vi "09 main.vi"() -> ()   [LabVIEW 2020]
panel:
  in  "Animate?":bool
  out "Unique visits":i32
  out "2D Picture":picture
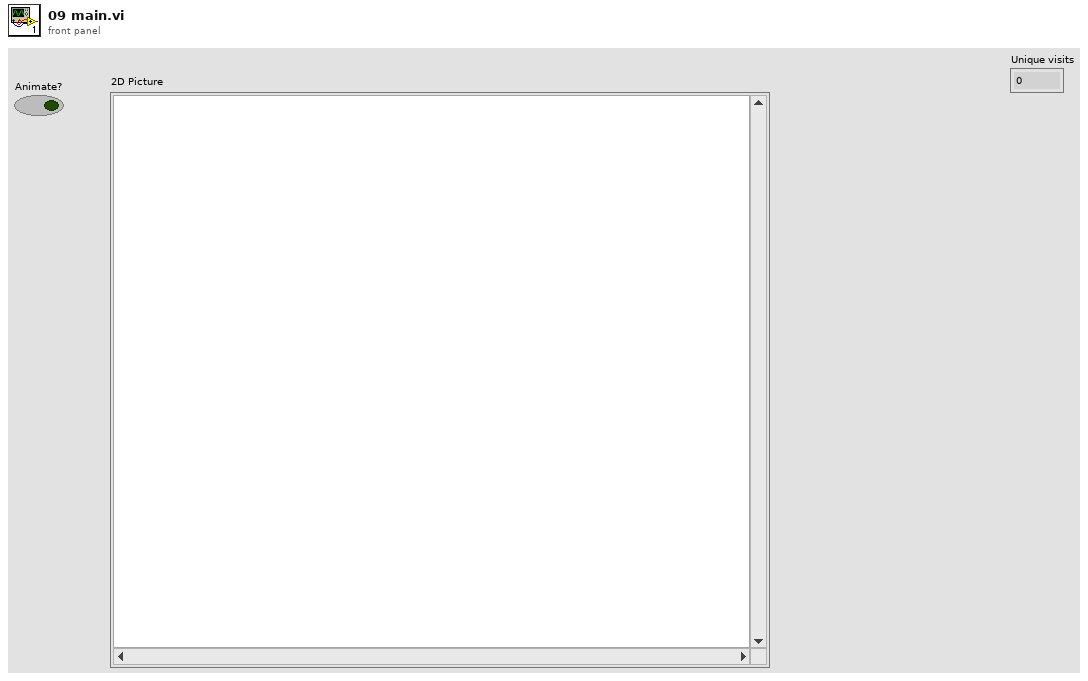
[diagram p1: front panel]
types:
  T1 = cluster{"left":i16, "top":i16, "right":i16, "bottom":i16}
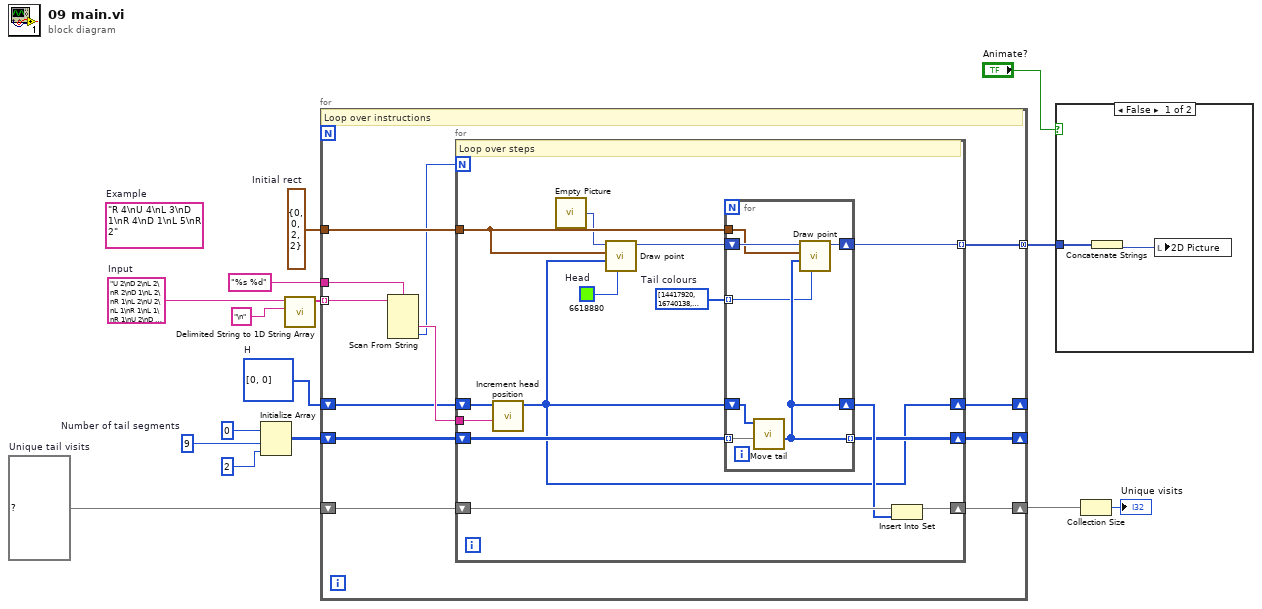
[diagram p0: block diagram]
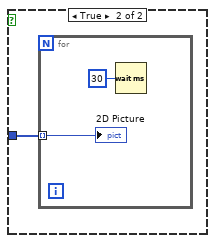
[diagram p2: hidden frame]
diagram:
  w12 = T1 {"left"=0, "top"=0, "right"=2, "bottom"=2}  # Initial rect
  w6 = 9  # Number of tail segments
  w11 = set{i32[]} {}  # Unique tail visits
  w8 = i32[] [0, 0]  # H
  w3 = "U 2\nD 2\nL 2\nR 2\nD 1\nL 2\nR 1\nL 2\nU 2\nL 1\nR 1\nL 1\nR 1\nU 2\nD 2\nL 1\nU 1\nL 2\nD 1\nU 2\nD 1\nR 1\nD 1\nU 2\nD 2\nU 1\nR 2\nD 2\nR 1\nU 1\nD 1\nR 1\nL 2\nU 2\nD 2\nL 1\nR 2\nL 2\nR 1\nD 1\nR 1\nD 2\nU 2\nR 2\nD 2\nU 2\nD 1\nU 1\nR 2\nU 2\nR 2\nU 2\nD 1\nU 1\nR 2\nD 1\nU 2\nL 1\nU 2\nD 1\nR 2\nU 1\nR 2\nD 1\nL 2\nR 1\nL 1\nR 2\nU 1\nL 1\nD 2\nL 2\nD 1\nR 2\nD 1\nR 2\nU 1\nD 1\nL 1\nR 1\nL 2\nR 1\nU 1\nD 2\nL 1\nD 2\nR 1\nL 1\nR 1\nU 2\nL 2\nD 1\nU 1\nD 2\nU 2\nR 2\nU 2\nR 1\nU 2\nD 1\nR 2\nD 2\nU 1\nD 1\nR 2\nU 1\nR 2\nL 1\nR 1\nD 2\nU 1\nR 3\nD 1\nR 1\nL 3\nD 2\nR 1\nD 1\nR 3\nL 2\nD 2\nL 1\nU 3\nD 3\nL 1\nD 1\nL 3\nD 1\nU 3\nL 1\nR 2\nU 2\nD 1\nL 2\nD 3\nR 1\nU 2\nL 2\nU 1\nL 1\nU 2\nD 2\nU 1\nL 1\nD 3\nR 1\nD 3\nR 1\nD 1\nU 1\nL 2\nU 3\nD 2\nU 1\nR 3\nD 1\nU 3\nL 3\nU 1\nR 2\nL 2\nR 1\nL 1\nU 1\nL 1\nD 2\nL 2\nU 2\nL 1\nD 2\nR 1\nU 2\nL 2\nR 2\nL 1\nU 2\nL 2\nR 3\nL 3\nD 1\nR 3\nL 3\nD 2\nU 3\nL 3\nD 2\nR 2\nL 2\nD 2\nU 2\nL 3\nR 1\nU 2\nL 1\nD 3\nU 2\nD 3\nL 2\nD 3\nU 1\nD 3\nU 3\nL 3\nD 2\nL 3\nR 2\nD 3\nR 1\nD 2\nU 2\nD 1\nU 3\nD 2\nL 2\nD 1\nR 1\nL 2\nR 2\nL 3\nU 3\nL 1\nD 2\nR 1\nL 2\nD 2\nR 1\nD 1\nL 4\nD 2\nR 3\nU 4\nR 4\nU 1\nD 4\nU 4\nD 4\nU 2\nR 3\nU 3\nR 4\nU 3\nL 2\nR 1\nU 4\nD 4\nR 2\nD 4\nR 2\nU 2\nD 1\nR 1\nL 3\nR 2\nD 3\nR 3\nU 1\nD 2\nR 4\nU 1\nD 4\nR 1\nU 1\nD 2\nU 4\nD 3\nL 1\nD 4\nL 2\nD 2\nR 3\nL 1\nU 4\nL 4\nU 3\nD 3\nL 2\nD 3\nU 1\nR 4\nD 3\nL 3\nD 4\nL 1\nD 2\nU 4\nL 2\nD 1\nR 3\nD 4\nU 3\nD 4\nU 2\nL 2\nR 3\nL 4\nR 2\nL 4\nU 3\nL 4\nD 3\nU 4\nL 2\nU 3\nR 2\nD 2\nU 1\nD 2\nL 1\nR 4\nD 3\nL 1\nD 3\nU 2\nL 4\nD 4\nL 4\nR 3\nL 3\nU 2\nL 1\nR 2\nL 4\nD 2\nL 3\nU 3\nD 1\nL 2\nR 3\nU 4\nR 1\nU 3\nD 4\nL 2\nU 2\nL 2\nR 5\nD 5\nU 3\nR 4\nL 4\nU 5\nD 3\nU 2\nL 5\nU 1\nR 3\nL 3\nU 4\nL 3\nD 5\nU 2\nR 1\nU 4\nR 5\nD 2\nL 1\nU 3\nR 5\nD 2\nU 3\nD 5\nU 2\nD 2\nU 2\nL 4\nU 5\nR 4\nU 4\nL 3\nU 5\nR 4\nL 4\nD 5\nR 4\nD 4\nL 2\nR 3\nL 5\nD 3\nU 2\nD 4\nR 1\nU 5\nR 4\nD 1\nU 1\nL 1\nU 3\nD 2\nU 4\nD 3\nU 5\nR 2\nU 5\nL 1\nR 5\nU 5\nR 4\nD 3\nR 1\nD 3\nU 3\nR 1\nL 1\nD 5\nU 4\nR 3\nD 3\nL 2\nU 1\nL 2\nU 5\nD 5\nU 2\nD 4\nL 2\nD 2\nL 1\nD 4\nU 2\nD 4\nR 1\nU 1\nD 4\nL 3\nD 3\nU 2\nD 2\nL 1\nD 5\nR 1\nL 2\nD 5\nU 5\nL 3\nD 1\nR 2\nL 2\nU 1\nL 2\nD 5\nL 1\nR 2\nD 4\nU 6\nL 4\nR 5\nD 4\nU 2\nR 1\nD 4\nL 2\nR 5\nL 6\nR 2\nU 6\nR 5\nD 1\nU 1\nL 6\nR 2\nL 6\nD 3\nL 2\nR 6\nU 6\nL 1\nD 3\nR 1\nD 2\nR 4\nL 4\nU 6\nL 3\nD 1\nU 1\nL 4\nR 3\nD 3\nR 6\nD 3\nL 4\nR 5\nL 5\nD 3\nU 3\nD 6\nR 4\nD 5\nL 2\nD 1\nR 4\nL 6\nR 5\nU 4\nD 5\nL 3\nD 1\nL 6\nD 5\nL 3\nU 3\nR 4\nL 4\nD 6\nR 3\nL 1\nR 1\nU 4\nD 6\nL 3\nR 2\nD 1\nL 2\nU 3\nD 3\nL 5\nU 6\nL 5\nD 5\nR 5\nU 6\nD 2\nU 2\nR 5\nU 6\nD 2\nR 1\nL 3\nU 1\nL 6\nU 1\nR 3\nL 3\nD 4\nU 2\nR 3\nL 1\nD 3\nR 5\nL 2\nD 3\nL 2\nU 6\nR 5\nU 5\nL 1\nU 5\nL 6\nD 4\nU 2\nL 5\nU 3\nD 2\nU 4\nD 4\nU 2\nR 5\nL 4\nD 3\nR 6\nD 1\nR 4\nU 5\nL 7\nD 2\nR 6\nU 4\nL 5\nD 5\nL 2\nD 1\nR 4\nD 6\nL 5\nD 4\nR 7\nU 4\nD 7\nU 4\nR 3\nL 7\nR 7\nD 3\nR 5\nU 2\nR 3\nD 5\nR 5\nU 4\nD 2\nU 5\nR 1\nU 5\nR 5\nU 7\nR 4\nD 6\nL 1\nU 3\nD 4\nU 3\nD 7\nU 2\nL 4\nD 6\nR 7\nU 1\nL 6\nD 4\nR 6\nD 4\nU 5\nL 4\nD 6\nL 5\nD 1\nL 5\nU 3\nL 3\nU 2\nR 6\nU 3\nD 4\nU 4\nL 1\nD 3\nL 3\nR 6\nU 2\nL 3\nD 7\nL 2\nU 7\nL 4\nU 4\nD 7\nL 4\nD 3\nL 3\nD 3\nU 1\nD 5\nL 1\nR 4\nD 7\nL 7\nD 6\nR 3\nU 1\nR 6\nL 4\nD 6\nR 5\nU 7\nL 6\nR 6\nL 3\nD 4\nU 1\nR 2\nL 1\nR 1\nU 4\nD 1\nL 4\nR 2\nU 4\nR 3\nD 1\nU 3\nR 4\nL 2\nU 4\nL 3\nD 7\nR 6\nU 4\nL 4\nD 7\nR 6\nD 7\nL 5\nR 5\nD 7\nR 4\nD 1\nL 6\nU 8\nL 4\nU 2\nL 6\nR 1\nL 5\nU 5\nD 3\nL 8\nR 3\nL 3\nR 5\nU 4\nR 6\nD 4\nU 1\nL 2\nR 8\nD 7\nU 3\nD 4\nL 8\nU 6\nL 5\nR 1\nU 1\nR 4\nU 5\nD 2\nR 2\nU 2\nL 1\nU 8\nD 4\nR 7\nU 3\nD 6\nR 6\nL 3\nR 8\nD 7\nU 2\nR 5\nL 3\nU 1\nD 6\nR 1\nD 3\nL 2\nU 2\nD 8\nU 8\nL 8\nU 5\nD 6\nU 6\nL 6\nU 6\nD 5\nR 8\nL 7\nD 6\nR 1\nD 4\nL 1\nU 7\nR 3\nL 2\nD 6\nR 6\nD 7\nL 6\nU 5\nR 4\nD 7\nU 7\nD 5\nL 4\nR 6\nD 3\nL 6\nU 2\nD 7\nR 7\nU 5\nD 3\nU 2\nL 1\nD 2\nU 4\nL 1\nR 3\nL 6\nU 9\nD 8\nL 3\nR 3\nD 4\nR 3\nU 6\nL 7\nD 8\nR 9\nD 1\nL 3\nR 6\nD 4\nL 3\nU 6\nL 7\nR 7\nU 9\nL 9\nR 7\nU 8\nR 7\nU 7\nD 1\nL 9\nR 6\nU 4\nD 6\nL 8\nR 7\nD 6\nU 5\nR 6\nD 8\nL 2\nD 5\nR 9\nU 9\nL 7\nU 2\nR 7\nL 6\nU 6\nD 5\nL 8\nD 7\nL 8\nD 9\nR 7\nL 5\nD 9\nL 7\nR 2\nL 6\nR 9\nD 8\nR 8\nU 7\nR 4\nL 6\nR 1\nU 9\nD 2\nR 7\nD 5\nR 4\nD 1\nU 7\nD 5\nR 4\nU 2\nD 5\nL 9\nR 6\nU 7\nD 5\nU 4\nD 6\nL 3\nR 6\nU 3\nR 9\nL 9\nU 4\nD 1\nU 3\nR 7\nD 8\nR 9\nU 1\nR 1\nU 4\nD 7\nR 1\nL 1\nR 8\nD 1\nU 1\nL 3\nU 2\nD 6\nR 6\nL 1\nR 9\nL 2\nD 3\nU 8\nD 9\nU 1\nL 10\nU 10\nD 8\nU 9\nL 3\nR 2\nD 3\nU 4\nL 2\nR 10\nL 9\nU 5\nL 5\nD 4\nL 7\nU 1\nL 1\nR 1\nL 7\nD 7\nU 7\nL 3\nU 10\nR 7\nU 9\nL 6\nR 2\nD 9\nL 10\nD 9\nL 9\nR 5\nL 5\nR 8\nD 9\nR 1\nD 6\nL 1\nU 9\nR 3\nL 10\nD 10\nL 5\nD 10\nR 3\nU 7\nD 6\nU 7\nD 3\nR 5\nD 5\nL 6\nD 4\nU 7\nD 7\nR 9\nU 10\nR 4\nU 1\nR 1\nU 8\nR 3\nU 10\nR 6\nL 1\nU 3\nR 9\nU 2\nD 8\nR 5\nD 3\nR 3\nU 9\nR 6\nL 8\nR 2\nL 5\nR 2\nL 10\nD 2\nL 3\nU 1\nD 10\nL 5\nR 10\nD 7\nL 2\nR 7\nU 6\nD 4\nL 8\nD 8\nU 3\nR 2\nU 10\nD 8\nU 7\nD 9\nU 4\nR 9\nL 2\nR 8\nU 9\nR 10\nU 10\nD 8\nR 8\nU 2\nL 7\nU 3\nL 1\nD 7\nR 1\nU 2\nR 8\nU 4\nD 4\nL 2\nU 9\nL 7\nD 7\nL 2\nR 2\nD 9\nL 11\nU 4\nL 3\nD 7\nU 7\nR 6\nD 7\nU 11\nR 4\nL 3\nR 2\nU 9\nL 1\nU 11\nD 7\nR 10\nD 10\nU 7\nL 1\nU 8\nL 2\nD 11\nL 6\nD 1\nL 8\nD 9\nU 9\nR 5\nL 4\nD 7\nU 8\nL 5\nD 3\nR 6\nL 5\nR 7\nL 7\nD 7\nL 10\nU 4\nL 1\nU 9\nD 2\nR 2\nU 4\nD 3\nR 9\nD 11\nU 10\nL 3\nR 9\nU 6\nL 1\nR 9\nL 8\nU 2\nL 3\nU 9\nD 2\nL 4\nD 5\nU 4\nL 5\nD 11\nL 6\nU 10\nD 9\nU 3\nL 9\nU 11\nD 3\nL 7\nD 4\nL 8\nU 5\nD 10\nL 7\nU 10\nL 10\nU 4\nD 10\nL 7\nR 2\nD 3\nL 6\nR 5\nU 11\nD 4\nU 6\nD 9\nR 2\nL 9\nU 9\nR 11\nU 9\nL 10\nR 8\nL 5\nR 2\nL 12\nR 8\nU 10\nR 7\nD 7\nU 3\nL 10\nU 10\nL 11\nU 1\nR 8\nD 4\nR 3\nD 7\nU 9\nL 2\nR 9\nL 8\nR 6\nL 7\nD 11\nU 12\nD 6\nU 7\nL 11\nD 1\nU 9\nR 7\nL 3\nD 3\nU 5\nR 5\nL 3\nR 11\nL 2\nU 9\nD 9\nR 8\nU 7\nD 5\nL 9\nD 2\nL 1\nR 5\nU 9\nR 10\nU 12\nL 9\nD 12\nR 5\nU 2\nL 7\nR 6\nL 1\nU 12\nL 10\nR 11\nD 1\nL 8\nU 6\nD 10\nR 10\nL 1\nU 11\nD 2\nR 6\nU 1\nR 4\nD 1\nR 6\nU 12\nD 1\nL 1\nU 4\nD 4\nU 12\nD 12\nL 5\nR 10\nD 4\nR 1\nD 8\nU 6\nR 7\nD 12\nU 9\nD 6\nU 6\nD 1\nR 2\nL 7\nR 5\nL 4\nU 1\nL 10\nR 8\nL 12\nD 11\nU 2\nL 10\nD 12\nR 9\nD 1\nU 7\nL 5\nD 4\nU 12\nL 12\nD 11\nU 11\nL 6\nD 2\nR 11\nL 1\nU 10\nL 12\nD 11\nR 8\nD 2\nL 10\nR 4\nL 10\nD 13\nL 10\nD 5\nU 9\nL 3\nD 2\nU 3\nD 11\nL 7\nD 11\nU 4\nD 11\nU 8\nL 5\nU 6\nL 3\nU 3\nR 8\nD 10\nR 1\nD 13\nL 7\nD 7\nR 1\nD 2\nL 3\nD 5\nR 5\nL 5\nU 7\nL 4\nD 1\nL 11\nR 10\nU 8\nD 9\nU 8\nR 11\nL 1\nR 6\nD 6\nU 4\nL 2\nD 11\nU 10\nD 4\nL 11\nR 5\nU 2\nD 10\nU 12\nL 12\nD 11\nL 12\nD 10\nL 4\nU 7\nD 1\nR 4\nL 10\nD 9\nR 5\nD 3\nL 3\nD 5\nR 9\nD 10\nL 8\nR 6\nD 4\nU 5\nR 11\nU 13\nR 10\nU 11\nR 9\nU 4\nD 8\nU 4\nD 6\nR 12\nU 12\nR 9\nU 12\nL 13\nU 6\nD 10\nR 2\nL 5\nU 3\nL 8\nR 11\nD 13\nR 6\nU 13\nL 3\nU 3\nD 4\nL 11\nU 14\nD 13\nU 1\nL 8\nU 13\nR 14\nU 2\nL 13\nR 1\nU 1\nL 13\nR 4\nD 10\nR 10\nD 14\nR 7\nD 10\nL 2\nR 7\nU 10\nR 13\nD 7\nU 11\nD 13\nL 7\nU 8\nL 4\nD 7\nL 2\nR 2\nL 7\nD 13\nU 2\nR 10\nU 2\nL 6\nR 11\nD 11\nL 13\nD 13\nL 14\nR 4\nL 7\nD 7\nR 11\nU 10\nD 3\nR 4\nL 2\nR 9\nU 7\nL 1\nR 5\nL 3\nU 8\nR 6\nU 10\nL 3\nR 12\nU 13\nD 3\nR 7\nD 1\nU 7\nR 13\nD 1\nR 10\nL 8\nR 8\nL 4\nR 9\nL 5\nD 13\nL 3\nU 8\nL 13\nU 4\nR 3\nU 2\nR 7\nD 9\nR 5\nU 4\nR 5\nD 7\nL 14\nR 13\nD 3\nL 12\nD 7\nU 5\nL 8\nD 10\nU 14\nD 8\nR 12\nU 3\nL 9\nR 7\nU 9\nR 5\nL 6\nU 13\nR 6\nL 8\nR 12\nD 13\nU 6\nL 12\nU 15\nD 10\nU 15\nD 7\nR 14\nD 5\nR 9\nU 11\nL 8\nD 9\nR 3\nU 3\nR 8\nD 6\nL 3\nR 9\nU 12\nL 12\nD 3\nU 13\nL 4\nR 3\nD 6\nR 12\nD 15\nL 3\nD 9\nR 9\nD 11\nL 6\nD 6\nL 3\nU 2\nD 6\nL 4\nD 3\nU 5\nD 1\nU 11\nR 11\nU 5\nL 12\nU 14\nR 1\nD 10\nL 8\nR 12\nL 5\nU 2\nD 2\nU 8\nD 5\nU 14\nD 2\nL 6\nR 5\nD 10\nL 10\nU 2\nR 2\nU 2\nL 15\nR 14\nD 12\nL 4\nU 2\nD 10\nR 14\nU 13\nR 9\nL 4\nU 15\nD 8\nR 4\nD 9\nU 1\nR 4\nD 3\nL 3\nD 7\nL 12\nR 8\nD 7\nL 15\nR 12\nU 10\nL 11\nR 1\nU 13\nR 14\nL 14\nD 14\nU 1\nR 1\nU 13\nL 15\nU 11\nD 15\nU 1\nR 15\nL 4\nU 12\nR 8\nU 10\nR 7\nU 3\nL 14\nU 14\nR 8\nD 1\nU 9\nL 3\nU 8\nD 5\nL 12\nU 15\nD 13\nL 11\nR 4\nU 12\nR 7\nL 15\nU 8\nD 7\nL 8\nR 7\nD 1\nL 12\nU 15\nL 15\nU 9\nR 10\nD 8\nU 10\nR 15\nD 3\nR 14\nD 13\nL 3\nR 2\nU 14\nL 3\nR 7\nL 15\nD 4\nR 14\nU 11\nL 2\nU 16\nL 6\nD 4\nL 3\nU 8\nR 16\nU 8\nD 13\nL 11\nU 11\nD 11\nR 14\nD 15\nL 4\nR 13\nU 4\nD 15\nU 10\nD 4\nR 14\nD 5\nU 7\nR 1\nL 6\nU 5\nL 10\nU 15\nL 14\nD 2\nU 5\nR 8\nL 14\nU 3\nR 9\nL 14\nR 8\nD 10\nL 8\nR 9\nL 14\nD 8\nR 16\nU 2\nD 12\nL 10\nR 12\nD 3\nR 11\nU 11\nD 7\nL 10\nD 15\nU 13\nR 5\nD 8\nU 12\nL 3\nR 6\nD 10\nR 5\nU 8\nR 16\nU 16\nD 3\nR 11\nD 7\nU 4\nR 14\nL 12\nU 5\nL 1\nU 14\nL 15\nR 13\nU 16\nD 6\nU 7\nD 11\nL 11\nU 13\nR 10\nD 16\nU 14\nL 1\nD 17\nU 14\nD 2\nL 17\nU 1\nL 6\nD 17\nR 13\nL 10\nU 16\nL 3\nU 4\nD 4\nL 2\nD 10\nL 2\nR 11\nL 14\nD 6\nU 13\nR 8\nD 8\nL 4\nU 8\nD 17\nR 11\nL 7\nU 15\nL 7\nR 11\nD 13\nU 3\nR 12\nD 9\nL 11\nD 14\nU 10\nL 11\nD 13\nL 17\nR 7\nD 4\nR 16\nD 1\nU 8\nL 6\nR 9\nL 7\nD 2\nL 3\nD 13\nL 6\nU 8\nL 13\nU 6\nL 12\nU 5\nD 1\nR 10\nL 17\nD 13\nU 1\nL 9\nR 8\nD 10\nU 10\nR 6\nU 17\nR 16\nD 3\nL 4\nD 13\nL 1\nU 6\nR 15\nU 6\nD 6\nU 1\nD 12\nU 12\nR 6\nD 2\nR 13\nD 16\nL 14\nD 16\nU 12\nR 13\nU 14\nR 4\nU 3\nD 3\nR 11\nU 2\nL 17\nR 13\nD 2\nR 5\nL 5\nD 17\nR 9\nD 3\nU 16\nR 8\nL 18\nR 12\nL 8\nR 10\nL 9\nR 4\nU 1\nD 4\nU 7\nL 2\nD 9\nR 12\nD 2\nR 1\nU 11\nD 4\nL 16\nU 18\nD 3\nR 14\nL 4\nU 2\nL 16\nR 4\nL 5\nD 3\nU 17\nR 3\nU 5\nR 8\nD 4\nL 3\nD 18\nL 12\nD 17\nU 15\nL 1\nD 17\nR 11\nU 5\nR 3\nL 16\nR 6\nL 14\nR 4\nU 15\nD 7\nR 15\nL 17\nU 14\nL 9\nR 9\nL 9\nD 11\nL 10\nU 7\nL 1\nU 11\nR 4\nU 7\nL 10\nD 16\nR 3\nL 17\nR 16\nL 9\nD 4\nR 17\nL 7\nU 5\nD 16\nR 5\nD 13\nU 5\nR 8\nD 10\nR 1\nL 2\nR 10\nU 12\nD 2\nU 12\nL 10\nR 6\nL 18\nU 7\nD 9\nR 16\nL 18\nD 17\nR 14\nU 9\nR 5\nD 4\nR 18\nD 6\nR 7\nU 12\nL 7\nD 11\nU 12\nR 12\nU 4\nL 8\nU 6\nD 11\nL 8\nR 18\nU 12\nR 2\nU 13\nD 3\nR 10\nD 4\nR 10\nL 18\nD 1\nL 18\nU 2\nD 19\nU 14\nL 14\nU 3\nD 14\nR 4\nL 10\nD 13\nR 6\nD 14\nR 13\nD 13\nR 11\nU 16\nL 18\nU 3\nR 8\nU 17\nR 7\nL 12\nD 3\nL 6\nR 6\nD 18\nL 2\nD 16\nR 1\nU 16\nR 14\nL 9\nD 6\nL 5\nD 6\nU 9\nL 11\nD 18\nR 5\nL 15\nD 18\nR 18\nL 3\nR 18\nL 18\nR 2\nL 15\nR 12\nD 9\nL 3\nU 17\nR 1\nU 18\nD 16\nU 17\nL 5\nU 9\nR 4\nL 14\nD 15\nR 11\nU 18\nL 19\nU 12\nR 13\nU 16\nD 16\nL 8\nD 16\nR 4\nU 5\nD 18\nR 13\nD 13\nU 9\nR 14\nL 14\nU 17\nD 9\nL 8\nR 18\nL 12\nR 16\nL 11\nU 14\nD 2\nL 19\nU 19\nD 11\nR 11\nU 16\nD 15\nU 16\nL 18\nD 3\nL 18\nU 7\nL 14\nD 6\nU 9\nD 2\nL 19\nD 17"  # Input
  (unwired) "R 4\nU 4\nL 3\nD 1\nR 4\nD 1\nL 5\nR 2"  # Example
  n1 = Initialize Array(0 ("Numeric"), w6, 2 ("dimension size")) -> (w5:i32[][])
  n2 = call <vilib>:"Delimited String to 1D String Array.vi"("delimiter"="\n", "delimited string"=w3) -> ("string array"=w14:string[])  [unwired: 9 in]
  n3 = for {
    tunnel: w14 -> [w27] mode=indexing
    tunnel: "%s %d" ("format string") -> [w26]
    shift-right: [w20] -> _
    shift-left: w8 -> [w24]
    tunnel: w12 -> [w22]
    shift-right: [w16] -> w10
    shift-left: w11 -> [w19]
    shift-right: [w18] -> _
    shift-left: w5 -> [w17]
    tunnel: [w23] -> w2 mode=concatenating
    # "Loop over instructions"
    n4 = Scan From String(format string=w26, input string=w27) -> (output 1=w25:string, output 2=w21:i32)  [unwired: 4 in, 3 out]
    n5 = for {
      N: w21 -> [_]
      tunnel: w25 -> [w29]
      tunnel: w22 -> [w34]
      shift-right: [w36] -> w20
      shift-left: w24 -> [w30]
      shift-right: [w37] -> w18
      shift-left: w17 -> [w39]
      shift-right: [w40] -> w16
      shift-left: w19 -> [w41]
      tunnel: [w31] -> w23 mode=indexing
      w32 = u32 6618880  # Head
      w33 = u32[] [14417920, 16740138, 16756736, 16771626, 5873408, 12124106, 65511, 13619455, 16716513]  # Tail colours
      # "Loop over steps"
      n6 = call "Increment head position.vi"("Direction"=w29, "H in"=w30) -> ("H out"=w36:i32[])  [unwired: 9 in]
      n7 = call "Empty Picture"() -> ("empty picture"=w28:picture)
      n8 = call "Draw point.vi"("color(black)"=w32, "Coordinate"=w36, "rect"=w34, "new picture in"=w28) -> ("new picture out"=w35:picture)  [unwired: 7 in]
      n9 = for {
        tunnel: w39 -> [w47] mode=indexing
        tunnel: [w44] -> w37 mode=indexing
        shift-right: [w44] -> w38
        shift-left: w36 -> [w48]
        tunnel: w34 -> [w43]
        shift-right: [w45] -> w31
        shift-left: w35 -> [w46]
        tunnel: w33 -> [w42] mode=indexing
        n10 = call "Move tail.vi"("T"=w47, "H"=w48) -> ("T 2"=w44:i32[])  [unwired: 9 in]
        n11 = call "Draw point.vi"("color(black)"=w42, "Coordinate"=w44, "rect"=w43, "new picture in"=w46) -> ("new picture out"=w45:picture)  [unwired: 7 in]
      }
      n12 = Insert Into Set(10:w38, 11:w41) -> (3:w40:set{i32[]})  [unwired: 1 out]
    }
  }
  n13 = case shown="False" "Animate?" {
    tunnel: w2 -> [w50 w51]
    frame False {
      n14 = Concatenate Strings(w50) -> (w49:picture)
      n15 = local write "2D Picture"(w49) -> ()
    }
    frame True {
      n16 = for {
        tunnel: w51 -> [w53] mode=indexing
        n17 = Wait (ms)(milliseconds to wait=u32 30) -> ()  [unwired: 1 out]
        "2D Picture" <- w53
      }
    }
  }
  n18 = Collection Size(1:w10) -> (0:→"Unique visits":i32)
